vi "Initiate (Continuous).vi"(7 "Enable Initiate Continuous (T: Enable)":bool=TRUE, 8 "error in (no error)":errorcluster, 11 "VISA resource name":refnum<visa-resource-name>) -> (0 "error out":errorcluster, 3 "VISA resource name out":refnum<visa-resource-name>)   [LabVIEW 2018, in "Agilent U2000 Series.lvlib"]
doc: "Sets the U2000 Series power sensor to be continuously initiated for either a single trigger cycle or continuous trigger cycles. A trigger cycle means that the U2000 Series power sensor exits the wait for trigger state and starts a measurement.\n\nThis VI usually appears in a pair, with Enable Initiate Continuous set to ON and OFF."
uses:
  Agilent U2000 Series.lvlib
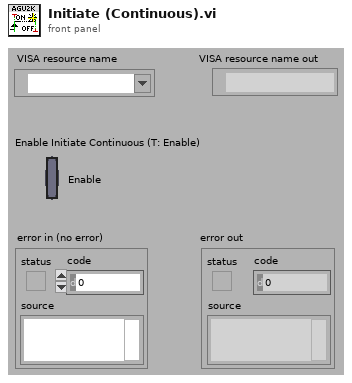
[diagram p1: front panel]
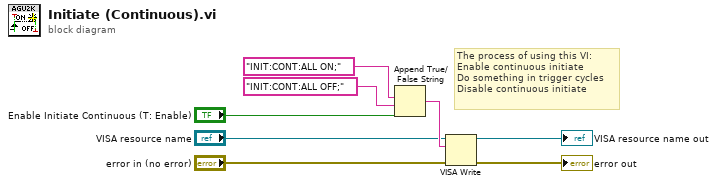
[diagram p0: block diagram]
diagram:
  # "The process of using this VI: \nEnable continuous initiate\nDo something in trigger cycles\nDisable continuous initiate"
  n1 = Append True/False String(1:"Enable Initiate Continuous (T: Enable)", 2:"INIT:CONT:ALL OFF;", 3:"INIT:CONT:ALL ON;") -> (0:w5:string)  [unwired: 1 out]
  n2 = VISA Write(VISA resource name="VISA resource name", write buffer=w5, error in (no error)="error in (no error)") -> (VISA resource name out=→"VISA resource name out":refnum<visa-resource-name>, error out=→"error out":errorcluster)  [unwired: 1 out]
